vi "Do.vi"(8 "error in (no error)":errorcluster, 10 "Actor in":refnum<class "Actor.lvclass">, 11 "Run Fan Msg":refnum<class "Run Fan Msg.lvclass">) -> (0 "error out":errorcluster, 2 "Actor out":refnum<class "Actor.lvclass">)   [LabVIEW 2018, in "Dual Fan.lvlib" / "Run Fan Msg.lvclass"]
uses:
  Run Fan Msg.lvclass
  <vilib>/ActorFramework/Actor/Actor.lvclass
  Dual Fan/Dual Fan.lvclass
  C:/Program Files (x86)/National Instruments/LabVIEW 2018/vi.lib/ActorFramework/Actor/Actor.lvclass
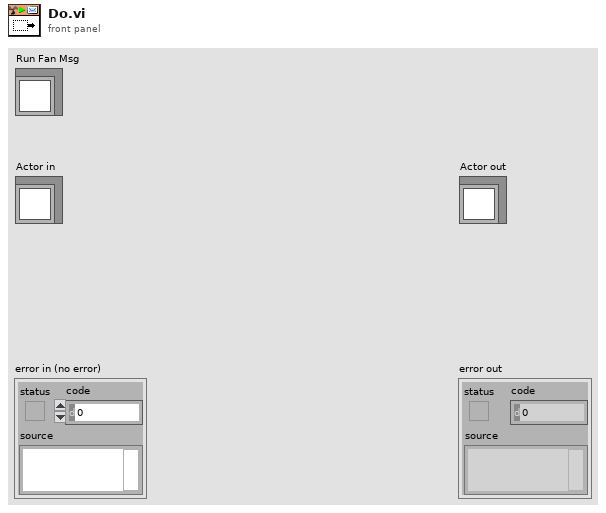
[diagram p1: front panel]
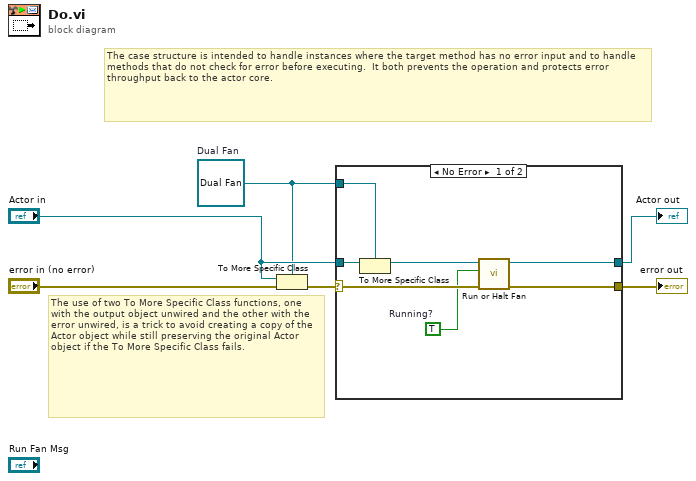
[diagram p0: block diagram]
diagram:
  w1 = refnum<class "Dual Fan.lvclass"> refnum  # Dual Fan
  # "The use of two To More Specific Class functions, one with the output object unwired and the other with the error unwired, is a trick to avoid creating a copy of the Actor object while still preserving the original Actor object if the To More Specific Class fails."
  # "The case structure is intended to handle instances where the target method has no error input and to handle methods that do not check for error before executing.  It both prevents the operation and protects error throughput back to the actor core."
  n1 = To More Specific Class(target class=w1, reference="Actor in", error in="error in (no error)") -> (error out=w5:errorcluster)  [unwired: 1 out]
  n2 = case shown="No Error" w5 {
    selector: w5 -> [w11 w15]
    tunnel: [w13 w15] -> w4
    tunnel: [w12 w14] -> w3
    tunnel: "Actor in" -> [w10 w14]
    tunnel: w1 -> [w9 _]
    frame No Error {
      w7 = TRUE  # Running?
      n3 = To More Specific Class(target class=w9, reference=w10) -> (specific class reference=w8:refnum<class "Dual Fan.lvclass">)  [unwired: 1 in, 1 out]
      n4 = call "Run or Halt Fan.vi"("error in (no error)"=w11, "Running?"=w7, "Dual Fan in"=w8) -> ("error out"=w13:errorcluster, "Dual Fan out"=w12:refnum<class "Dual Fan.lvclass">)  [unwired: 7 in]
    }
    frame Error {
      # "If type check fails, pass the original object out again."
    }
  }
  "error out" <- w4
  "Actor out" <- w3
